vi "Actor Core.vi"(8 "error in":errorcluster, 11 "CANopen Actor in":refnum<class "CANopen Actor.lvclass">) -> (0 "error out":errorcluster, 3 "Actor out":refnum<class "Actor.lvclass">)   [LabVIEW 2024, in "CANopen Actor.lvlib" / "CANopen Actor.lvclass"]
doc: "<p>(<strong>Filename</strong>: <span class=\"dnl\">Actor Framework.lvlib:Actor.lvclass:Actor Core.vi</span>)</p>\n<p>Receives messages to the actor, reacts to them, and initiates any error handling that may shut the actor down.</p>\n<p>Descendant classes may override this VI to append parallel tasks for the actor to complete while it handles messages. Overrides use the <a href=\"nihelplauncher://docs/csh?context=lvcore_glang_udclass\">Call Parent Class Method</a> node.</p>"
uses:
  CANopen Actor.lvclass
  CANopen Actor.lvclass/CANopen Actor.ctl
  <vilib>/ActorFramework/Actor/Actor.lvclass
  CANopen/CAN Task/CAN Task/CANopen Task Actor.lvclass
  CANopen/CAN Task/CANopen Task Actor Messages/Start Msg/Start Msg.lvclass
  C:/Program Files/National Instruments/LabVIEW 2024/vi.lib/ActorFramework/Actor/Actor.lvclass
  D:/git/CANopen-XNET/CANopen/CAN Task/CAN Task/CANopen Task Actor.lvclass
  D:/git/CANopen-XNET/CANopen Actor/CANopen Actor/CANopen Actor.lvclass
  D:/git/CANopen-XNET/CANopen Actor Interface/CANopen Actor Interface/CANopen Actor Interface.lvclass
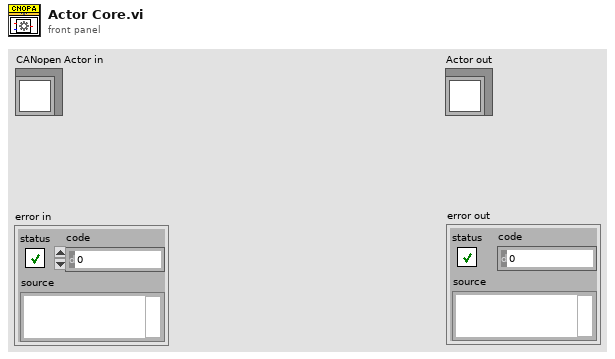
[diagram p1: front panel]
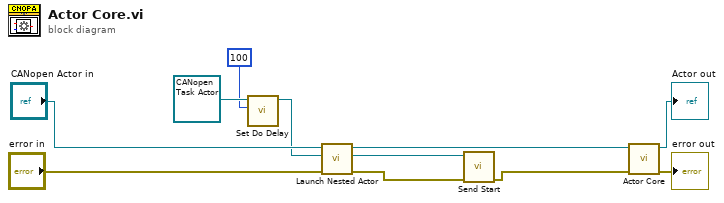
[diagram p0: block diagram]
diagram:
  n1 = call "Set Do Delay.vi"("Do Delay"=100, "CAN Task in"=refnum<class "CANopen Task Actor.lvclass"> refnum ("CAN Task.lvlib:CAN Task.lvclass")) -> ("CAN Task out"=w2:refnum<class "CANopen Task Actor.lvclass">)  [unwired: 9 in]
  n2 = call <vilib>:"Launch Nested Actor.vi"("error in (no error)"="error in", "Nested Actor"=w2, "Caller Actor in"="CANopen Actor in") -> ("error out"=w4:errorcluster, "Nested Actor's Enqueuer"=w5:refnum<class "Message Enqueuer.lvclass">, "Caller Actor out"=w7:refnum<class "CANopen Actor.lvclass">)  [unwired: 6 in]
  n3 = call "Send Start.vi"("error in (no error)"=w4, "Message Enqueuer"=w5) -> ("error out"=w3:errorcluster)  [unwired: 8 in, 1 out]
  n4 = call-parent "Actor Core.vi"("error in"=w3, "Actor in"=w7) -> ("error out"=→"error out":errorcluster, "Actor out"=→"Actor out":refnum<class "Actor.lvclass">)  [unwired: 8 in]
